vi "sub Menu open file.vi"(8 "error in (no error)":errorcluster, 11 "LF2R IDE in":refnum<class "LF2R IDE.lvclass">) -> (0 "error out":errorcluster, 3 "LF2R IDE out":refnum<class "LF2R IDE.lvclass">)   [LabVIEW 2018, in "LF2R IDE.lvlib" / "LF2R IDE.lvclass"]
uses:
  LF2R IDE.lvclass
  LF2R IDE.lvclass/LF2R IDE.ctl
  ScintillaNET/ScintillaNET.lvclass
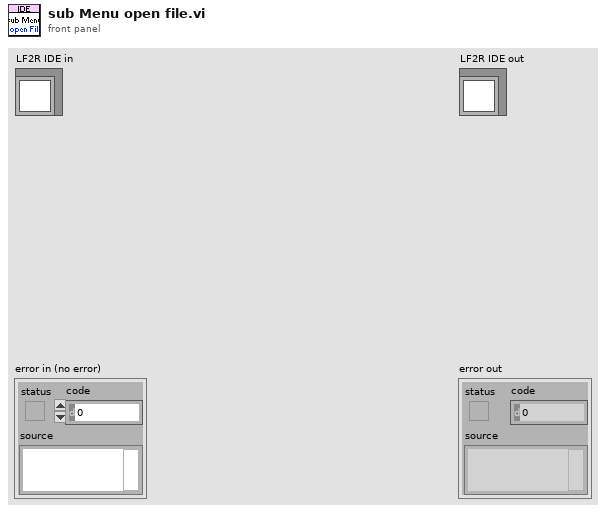
[diagram p1: front panel]
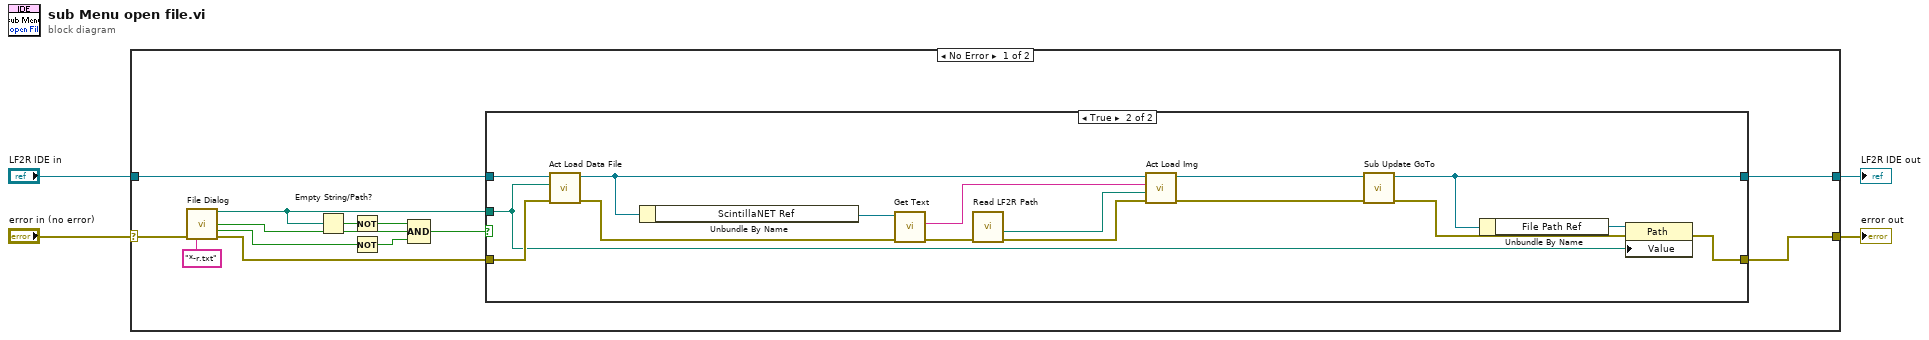
[diagram p0: block diagram]
diagram:
  n1 = case shown="No Error" "error in (no error)" {
    selector: "error in (no error)" -> [w6 w37]
    tunnel: [w15 w37] -> w3
    tunnel: [w16 w36] -> w1
    tunnel: "LF2R IDE in" -> [w17 w36]
    frame No Error {
      n2 = call "File Dialog"("error in"=w6, "pattern (all files)"="*-r.txt" ("pattern label")) -> ("selected path"=w8:path, "exists"=w11:bool, "cancelled"=w14:bool, "error out"=w7:errorcluster)  [unwired: 10 in]
      n3 = Empty String/Path?(string/path=w8) -> (empty?=w13:bool)
      n4 = Not(x=w13) -> (.not. x?=w12:bool)
      n5 = Not(x=w14) -> (.not. x?=w10:bool)
      n6 = Compound Arithmetic op=AND(w12, w11, w10) -> (w9:bool)
      n7 = case shown="True" w9 {
        tunnel: [w19 w29] -> w16
        tunnel: [w18 w32] -> w15
        tunnel: w17 -> [w19 w35]
        tunnel: w8 -> [_ w33]
        tunnel: w7 -> [w18 w34]
        frame False {
        }
        frame True {
          n8 = call "Act Load Data File.vi"("error in (no error)"=w34, "File Path"=w33, "IDE simple in"=w35) -> ("error out"=w21:errorcluster, "IDE simple out"=w23:refnum<class "LF2R IDE.lvclass">)  [unwired: 7 in]
          n9 = Unbundle By Name(w23) -> ("ScintillaNET Ref"=w24:refnum<class "ScintillaNET.lvclass">)
          n10 = call "Get Text.vi"("error in (no error)"=w21, "ScintillaNET in"=w24) -> ("error out"=w22:errorcluster, "Text"=w20:string)  [unwired: 7 in, 1 out]
          n11 = call "Read LF2R Path.vi"("error in (no error)"=w22) -> ("error out"=w27:errorcluster, "PNG Path"=w28:path)  [unwired: 6 in, 3 out]
          n12 = call "Act Load Img.vi"("error in (no error)"=w27, "PNG Path"=w28, "File String"=w20, "LF2R IDE in"=w23) -> ("error out"=w25:errorcluster, "LF2R IDE out"=w26:refnum<class "LF2R IDE.lvclass">)  [unwired: 6 in]
          n13 = call "Sub Update GoTo.vi"("error in (no error)"=w25, "LF2R IDE in"=w26) -> ("error out"=w31:errorcluster, "LF2R IDE out"=w29:refnum<class "LF2R IDE.lvclass">)  [unwired: 8 in]
          n14 = Unbundle By Name(w29) -> ("File Path Ref"=w30:refnum<vi>)
          n15 = property class="Path"(reference=w30, error in=w31, "Value"=w33) -> (error out=w32:errorcluster)  [unwired: 1 out]
        }
      }
    }
    frame Error {
    }
  }
  "error out" <- w3
  "LF2R IDE out" <- w1
